vi "initialize_dcs.vi"(8 "error in (no error)":errorcluster) -> (0 "error out":errorcluster, 2 "Dust Spot Array":T1[](array[typedef]), 3 "Dust Point Array":T2[](array[typedef]))   [LabVIEW 2013]
doc: "Initializes DCS with the last 25 rows from dcs_points and dcs_spot."
uses:
  User Interface/Controls/dcs points.ctl
  User Interface/Controls/dcs_spot.ctl
  <vilib>/addons/database/_DB Variant To Data/Database Variant To Data.xnode
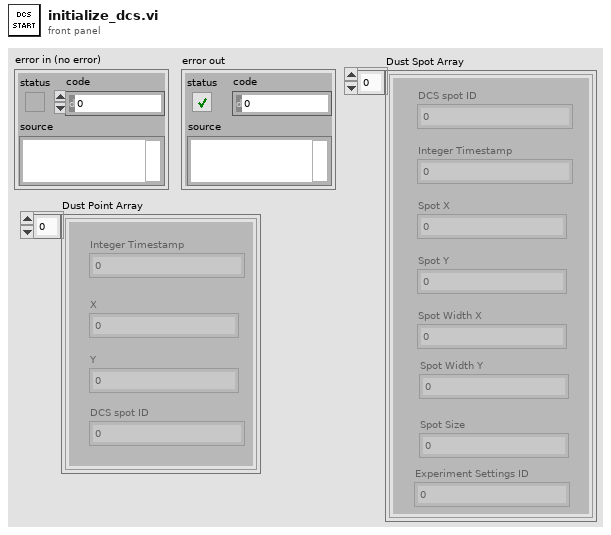
[diagram p1: front panel]
types:
  T1 = typedef "dcs_spot.ctl" = cluster{"DCS spot ID":i32, "Integer Timestamp":i64, "Spot X":dbl, "Spot Y":dbl, "Spot Width X":dbl, "Spot Width Y":dbl, "Spot Size":i32, "Experiment Settings ID":i32}
  T2 = typedef "dcs points.ctl" = cluster{"Integer Timestamp":i64, "X":dbl, "Y":dbl, "DCS spot ID":i32}
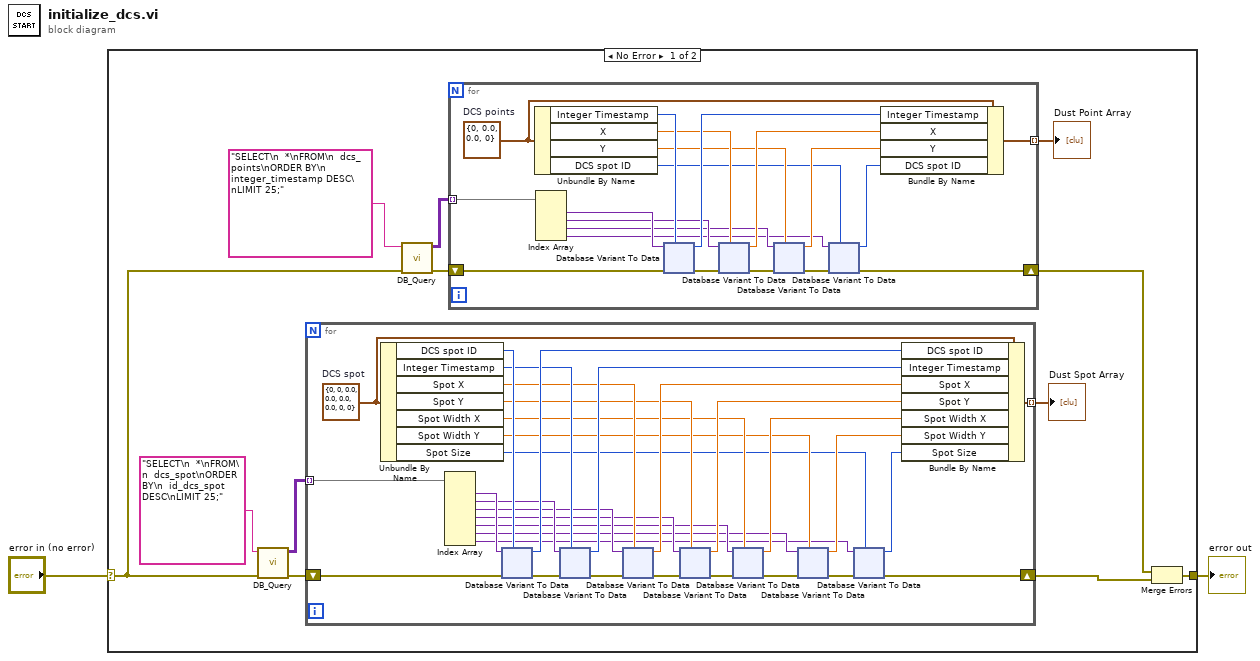
[diagram p0: block diagram]
diagram:
  n1 = case shown="No Error" "error in (no error)" {
    selector: "error in (no error)" -> [w3 w419]
    tunnel: [w12 w419] -> w1
    frame No Error {
      n2 = call "DB_Query.vi"("error in (no error)"=w3, "Parameterized Query"="SELECT\n  *\nFROM\n  dcs_spot\nORDER BY\n  id_dcs_spot DESC\nLIMIT 25;" ("SQL query")) -> ("error out"=w5:errorcluster, "Results"=w6:variant[][])  [unwired: 7 in, 1 out]
      n3 = for {
        tunnel: w6 -> [w194] mode=indexing
        shift-right: [w166] -> w7
        shift-left: w5 -> [w191]
        tunnel: [w193] -> w13 mode=indexing
        w192 = T1 {"DCS spot ID"=0, "Integer Timestamp"=0, "Spot X"=0.0, "Spot Y"=0.0, "Spot Width X"=0.0, "Spot Width Y"=0.0, "Spot Size"=0, "Experiment Settings ID"=0}  # DCS spot
        n4 = Unbundle By Name(w192) -> ("DCS spot ID"=w190:i32, "Integer Timestamp"=w185:i64, "Spot X"=w182:dbl, "Spot Y"=w177:dbl, "Spot Width X"=w173:dbl, "Spot Width Y"=w169:dbl, "Spot Size"=w164:i32)
        n5 = Index Array(array=w194) -> (element #1=w189:variant, element #2=w186:variant, element #3=w183:variant, element #4=w178:variant, element #5=w174:variant, element #6=w170:variant, element #7=w165:variant)  [unwired: 7 in]
        n6 = xnode "Database Variant To Data"("database variant"=w189, "error in (no error)"=w191, "type"=w190) -> ("data"=w188:i32, "error out"=w187:errorcluster)
        n7 = xnode "Database Variant To Data"("database variant"=w186, "error in (no error)"=w187, "type"=w185) -> ("data"=w184:i64, "error out"=w180:errorcluster)
        n8 = xnode "Database Variant To Data"("database variant"=w183, "error in (no error)"=w180, "type"=w182) -> ("data"=w181:dbl, "error out"=w179:errorcluster)
        n9 = xnode "Database Variant To Data"("database variant"=w178, "error in (no error)"=w179, "type"=w177) -> ("data"=w176:dbl, "error out"=w175:errorcluster)
        n10 = xnode "Database Variant To Data"("database variant"=w174, "error in (no error)"=w175, "type"=w173) -> ("data"=w172:dbl, "error out"=w171:errorcluster)
        n11 = xnode "Database Variant To Data"("database variant"=w170, "error in (no error)"=w171, "type"=w169) -> ("data"=w168:dbl, "error out"=w167:errorcluster)
        n12 = xnode "Database Variant To Data"("database variant"=w165, "error in (no error)"=w167, "type"=w164) -> ("data"=w163:i32, "error out"=w166:errorcluster)
        n13 = Bundle By Name(cluster=w192, "DCS spot ID"=w188, "Integer Timestamp"=w184, "Spot X"=w181, "Spot Y"=w176, "Spot Width X"=w172, "Spot Width Y"=w168, "Spot Size"=w163) -> (w193:T1)
      }
      "Dust Spot Array" <- w13
      n14 = call "DB_Query.vi"("error in (no error)"=w3, "Parameterized Query"="SELECT\n  *\nFROM\n  dcs_points\nORDER BY\n  integer_timestamp DESC\nLIMIT 25;" ("format string")) -> ("error out"=w11:errorcluster, "Results"=w10:variant[][])  [unwired: 7 in, 1 out]
      n15 = for {
        tunnel: w10 -> [w34] mode=indexing
        shift-right: [w21] -> w8
        shift-left: w11 -> [w28]
        tunnel: [w33] -> w14 mode=indexing
        w31 = T2 {"Integer Timestamp"=0, "X"=0.0, "Y"=0.0, "DCS spot ID"=0}  # DCS points
        n16 = Unbundle By Name(w31) -> ("Integer Timestamp"=w30:i64, "X"=w25:dbl, "Y"=w19:dbl, "DCS spot ID"=w16:i32)
        n17 = Index Array(array=w34) -> (element #1=w32:variant, element #2=w26:variant, element #3=w20:variant, element #4=w17:variant)  [unwired: 4 in]
        n18 = xnode "Database Variant To Data"("database variant"=w32, "error in (no error)"=w28, "type"=w30) -> ("data"=w29:i64, "error out"=w27:errorcluster)
        n19 = xnode "Database Variant To Data"("database variant"=w26, "error in (no error)"=w27, "type"=w25) -> ("data"=w24:dbl, "error out"=w23:errorcluster)
        n20 = xnode "Database Variant To Data"("database variant"=w20, "error in (no error)"=w23, "type"=w19) -> ("data"=w18:dbl, "error out"=w22:errorcluster)
        n21 = xnode "Database Variant To Data"("database variant"=w17, "error in (no error)"=w22, "type"=w16) -> ("data"=w15:i32, "error out"=w21:errorcluster)
        n22 = Bundle By Name(cluster=w31, "Integer Timestamp"=w29, "X"=w24, "Y"=w18, "DCS spot ID"=w15) -> (w33:T2)
      }
      "Dust Point Array" <- w14
      n23 = Merge Errors(w8, w7) -> (w12:errorcluster)
    }
    frame Error {
    }
  }
  "error out" <- w1
